vi "Void Code Block.vi"(8 "Error In":errorcluster, 11 "Code":string) -> (0 "Error Out":errorcluster)   [LabVIEW 2014, in "Arduino Extra Functions.lvlib"]
uses:
  <vilib>/Aledyne-TSXperts/Arduino Compatible Compiler for LabVIEW/addons/Arduino Extra Functions/Arduino Extra Functions.lvlib
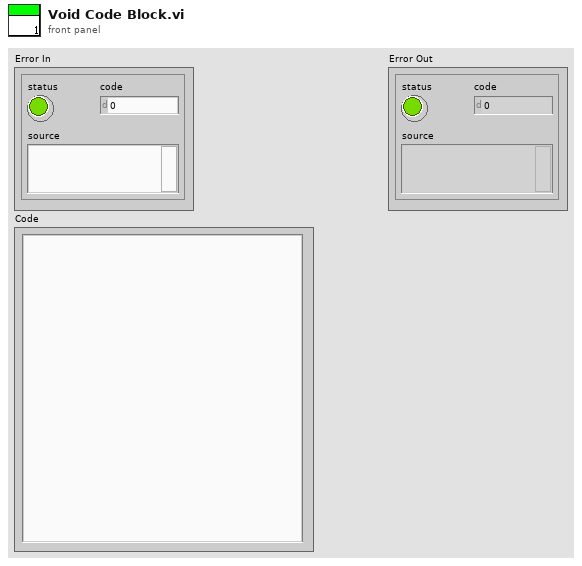
[diagram p1: front panel]
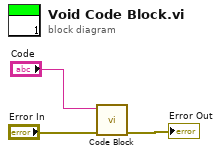
[diagram p0: block diagram]
diagram:
  n1 = call <vilib>:"Code Block.vi"("Error In"="Error In", "Code"="Code") -> ("Error Out"=→"Error Out":errorcluster)  [unwired: 9 in]
